vi "VmaxVmin notifier.vi"(8 "error in (no error)":errorcluster) -> (0 "error out":errorcluster, 9 "VmaxVmin Range":string, 10 "Channel":string)   [LabVIEW 2015]
uses:
  DAQ Engine VIs/PXI Globals.vi
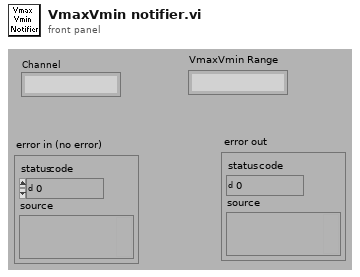
[diagram p1: front panel]
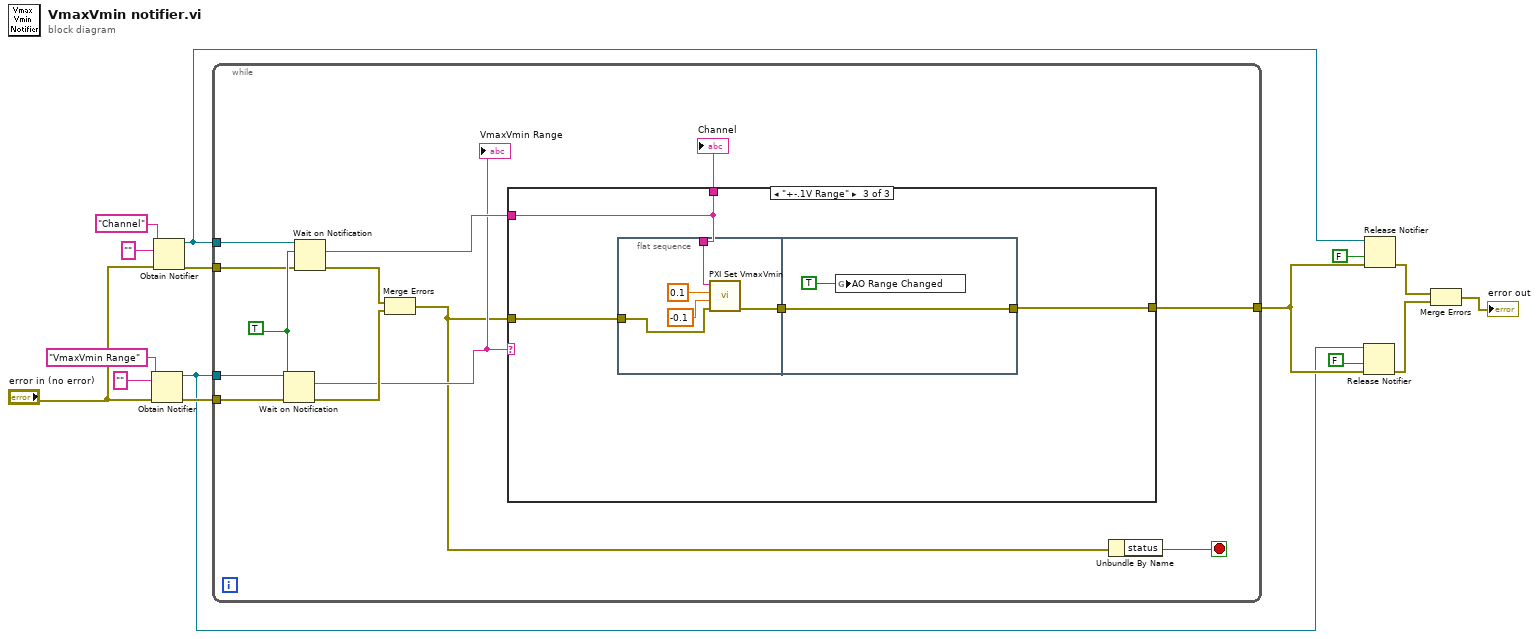
[diagram p0: block diagram]
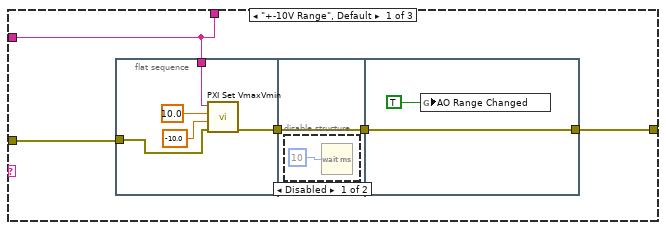
[diagram p2: hidden frame]
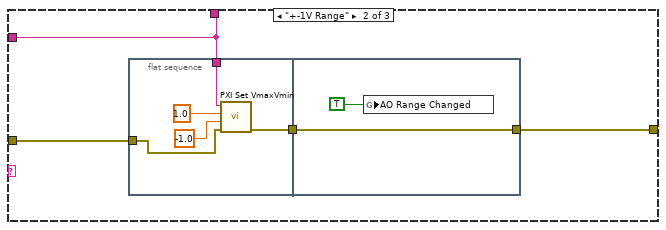
[diagram p4: hidden frame]
diagram:
  n1 = Obtain Notifier(name (unnamed)="VmaxVmin Range" ("Notifier Name 2"), notification data type="", error in (no error)="error in (no error)") -> (notifier out=w3:refnum<notifier>, error out=w4:errorcluster)  [unwired: 1 in, 1 out]
  n2 = Obtain Notifier(name (unnamed)="Channel", notification data type="", error in (no error)="error in (no error)") -> (notifier out=w2:refnum<notifier>, error out=w5:errorcluster)  [unwired: 1 in, 1 out]
  n3 = while {
    tunnel: [w27] -> w6
    tunnel: w2 -> [w24]
    tunnel: w3 -> [w23]
    tunnel: w5 -> [w22]
    tunnel: w4 -> [w21]
    stop <- w17 stop-if-true
    w25 = TRUE
    n4 = Wait on Notification(notifier=w23, ignore previous (F)=w25, error in (no error)=w21) -> (notification=w18:string, error out=w19:errorcluster)  [unwired: 1 in, 2 out]
    "VmaxVmin Range" <- w18
    n5 = Wait on Notification(notifier=w24, ignore previous (F)=w25, error in (no error)=w22) -> (notification=w26:string, error out=w20:errorcluster)  [unwired: 1 in, 2 out]
    n6 = Merge Errors(w20, w19) -> (w16:errorcluster)
    n7 = case shown="\"+-.1V Range\"" w18 {
      tunnel: [w32 w45 w56] -> w28
      tunnel: w16 -> [w33 w43 w54]
      tunnel: [w31 w44 w55] -> w27
      tunnel: w26 -> [w32 w45 w56]
      frame "+-10V Range", Default {
        n8 = flat-sequence {
          tunnel: w32 -> [w36]
          tunnel: [w35] -> w30
          tunnel: w33 -> [w34]
          tunnel: w30 -> [w39]
          tunnel: [w39] -> w29
          tunnel: w29 -> [w42]
          tunnel: [w42] -> w31
          frame #0 {
            n9 = call "PXI Set VmaxVmin.vi"("error in (no error)"=w34, "Vmin"=-10.0, "Vmax"=10.0, "channel"=w36) -> ("error out"=w35:errorcluster)  [unwired: 5 in]
          }
          frame #1 {
            n10 = disable-structure shown="Disabled" {
              frame Disabled {
                n11 = Wait (ms)(milliseconds to wait=10) -> ()  [unwired: 1 out]
              }
              frame Enabled {
              }
            }
          }
          frame #2 {
            n12 = global write "PXI Globals.vi" "AO Range Changed"(TRUE) -> ()
          }
        }
      }
      frame "+-1V Range" {
        n13 = flat-sequence {
          tunnel: [w49] -> w46
          tunnel: w45 -> [w47]
          tunnel: w43 -> [w48]
          tunnel: w46 -> [w53]
          tunnel: [w53] -> w44
          frame #0 {
            n14 = call "PXI Set VmaxVmin.vi"("error in (no error)"=w48, "Vmin"=-1.0, "Vmax"=1.0, "channel"=w47) -> ("error out"=w49:errorcluster)  [unwired: 5 in]
          }
          frame #1 {
            n15 = global write "PXI Globals.vi" "AO Range Changed"(TRUE) -> ()
          }
        }
      }
      frame "+-.1V Range" {
        n16 = flat-sequence {
          tunnel: w56 -> [w60]
          tunnel: [w59] -> w57
          tunnel: w54 -> [w58]
          tunnel: w57 -> [w64]
          tunnel: [w64] -> w55
          frame #0 {
            n17 = call "PXI Set VmaxVmin.vi"("error in (no error)"=w58, "Vmin"=-0.1, "Vmax"=0.1, "channel"=w60) -> ("error out"=w59:errorcluster)  [unwired: 5 in]
          }
          frame #1 {
            n18 = global write "PXI Globals.vi" "AO Range Changed"(TRUE) -> ()
          }
        }
      }
    }
    "Channel" <- w28
    n19 = Unbundle By Name(w16) -> ("status"=w17:bool)
  }
  n20 = Release Notifier(notifier=w3, force destroy? (F)=FALSE, error in (no error)=w6) -> (error out=w10:errorcluster)  [unwired: 2 out]
  n21 = Release Notifier(notifier=w2, force destroy? (F)=FALSE, error in (no error)=w6) -> (error out=w9:errorcluster)  [unwired: 2 out]
  n22 = Merge Errors(w9, w10) -> (→"error out":errorcluster)
